vi "Set DC Bias.vi"(7 "error in":errorcluster {"code" format="%.0x"}, 9 "Assign  DC bias according to the chart on the right":dbl=4.0, 10 "VISA resource name":refnum<visa-resource-name>="GPIB12::28::INSTR") -> (0 "error out":errorcluster {"code" format="%.0x"}, 1 "Send string":string, 2 "Read out result":string, 3 "VISA resource name out":refnum<visa-resource-name>)   [LabVIEW 2016, in "AH2500A.lvclass"]
uses:
  SMOs/AH2500A/AH2500A.lvclass
panel:
  in  "byte count":u32=128
  # "DC bias enable setting"
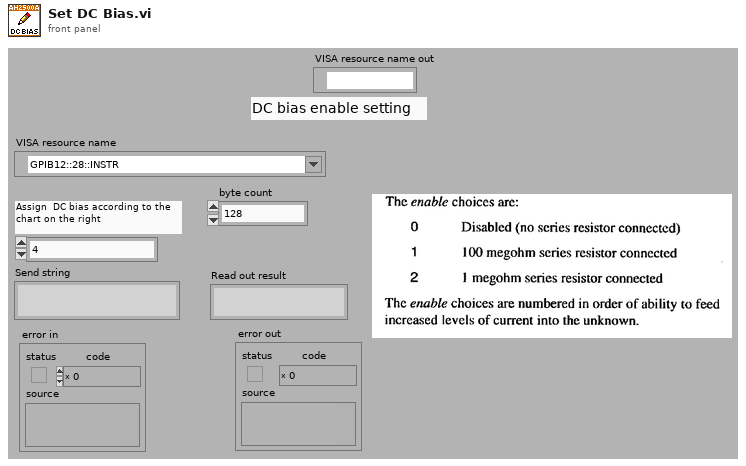
[diagram p1: front panel]
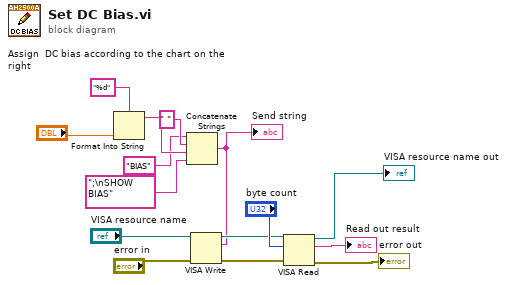
[diagram p0: block diagram]
diagram:
  n1 = Format Into String(format string="%d", "Assign  DC bias according to the chart on the right") -> (resulting string=w11:string)  [unwired: 2 in, 1 out]
  n2 = Concatenate Strings("BIAS" ("string"), " " ("string"), w11, ";\nSHOW BIAS" ("format string")) -> (w4:string)
  "Send string" <- w4
  n3 = VISA Write(VISA resource name="VISA resource name", write buffer=w4, error in (no error)="error in") -> (VISA resource name out=w7:refnum<visa-resource-name>, error out=w6:errorcluster)  [unwired: 1 out]
  n4 = VISA Read(VISA resource name=w7, byte count="byte count", error in (no error)=w6) -> (VISA resource name out=→"VISA resource name out":refnum<visa-resource-name>, read buffer=→"Read out result":string, error out=→"error out":errorcluster)  [unwired: 1 out]
